vi "Show UI For Selection.vi"(8 "Error In":errorcluster, 11 "Pane Relief Main UI in":refnum<class "Pane Relief Main UI.lvclass">) -> (0 "Error Out":errorcluster, 3 "Pane Relief Main UI out":refnum<class "Pane Relief Main UI.lvclass">)   [LabVIEW 2017, in "Pane Relief Main UI.lvlib" / "Pane Relief Main UI.lvclass"]
uses:
  Pane Relief Main UI.lvclass
  Pane Relief Main UI.lvclass/Pane Relief Main UI.ctl
  Panel Object Actions UI/Panel Object Actions UI Messages/Show Panel Object Actions UI Msg/Show Panel Object Actions UI Msg.lvclass/Show Panel Object Actions UI Msg.ctl
  <vilib>/ActorFramework/Message Enqueuer/Message Enqueuer.lvclass/Message Enqueuer.ctl
  <vilib>/ActorFramework/Message Enqueuer/Enqueue.vi
  Panel Object Actions UI/Panel Object Actions UI Messages/Show Panel Object Actions UI Msg/Show Panel Object Actions UI Msg.lvclass
  C:/Program Files (x86)/National Instruments/LabVIEW 2017/vi.lib/ActorFramework/Message/Message.lvclass
  <vilib>/ActorFramework/Message Priority Queue/Priority Enqueue.vi
  Panel Object/Panel Object.lvclass
  <vilib>/MNProjects/Panel Manager/panel-actors/Source/Panel Actor Messages/Show Panel Msg/Show Panel Msg.lvclass
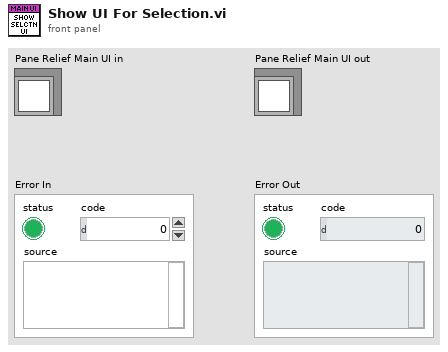
[diagram p1: front panel]
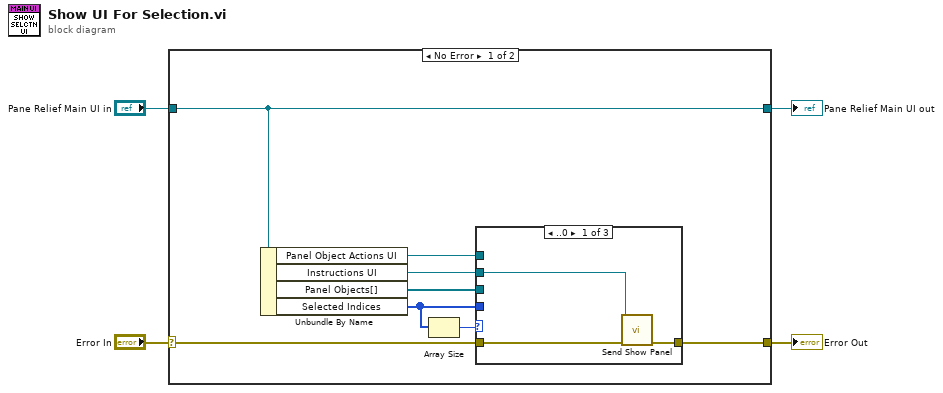
[diagram p0: block diagram]
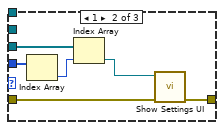
[diagram p2: hidden frame]
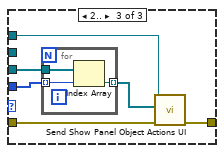
[diagram p3: hidden frame]
diagram:
  n1 = case shown="No Error" "Error In" {
    selector: "Error In" -> [w10 w32]
    tunnel: [w9 w32] -> w1
    tunnel: [w11 w31] -> w3
    tunnel: "Pane Relief Main UI in" -> [w11 w31]
    frame No Error {
      n2 = Unbundle By Name(w11) -> ("Panel Object Actions UI"=w6:refnum<class "Message Enqueuer.lvclass">, "Instructions UI"=w7:refnum<class "Message Enqueuer.lvclass">, "Panel Objects[]"=w12:refnum<class "Panel Object.lvclass">[], "Selected Indices"=w5:i32[])
      n3 = Array Size(array=w5) -> (size(s)=w8:i32)
      n4 = case shown="..0" w8 {
        tunnel: w12 -> [_ w21 w24]
        tunnel: w10 -> [w14 w19 w26]
        tunnel: [w15 w18 w27] -> w9
        tunnel: w7 -> [w13 _ _]
        tunnel: w6 -> [_ _ w25]
        tunnel: w5 -> [_ w17 w22]
        frame ..0 {
          n5 = call <vilib>:"Send Show Panel.vi"("error in (no error)"=w14, "Message Enqueuer in"=w13) -> ("error out"=w15:errorcluster)  [unwired: 8 in, 1 out]
        }
        frame 1 {
          n6 = Index Array(array=w17) -> (element=w16:i32)  [unwired: 1 in]
          n7 = Index Array(array=w21, index=w16) -> (element=w20:refnum<class "Panel Object.lvclass">)
          n8 = call-dynamic "Show Settings UI.vi"("Error In"=w19, "Panel Object in"=w20) -> ("Error Out"=w18:errorcluster)  [unwired: 8 in, 1 out]
        }
        frame 2.. {
          n9 = for {
            tunnel: w24 -> [w30]
            tunnel: [w29] -> w23 mode=indexing
            tunnel: w22 -> [w28] mode=indexing
            n10 = Index Array(array=w30, index=w28) -> (element=w29:refnum<class "Panel Object.lvclass">)
          }
          n11 = call "Send Show Panel Object Actions UI.vi"("error in (no error)"=w26, "Panel Objects"=w23, "Message Enqueuer"=w25) -> ("error out"=w27:errorcluster)  [unwired: 7 in, 1 out]
        }
      }
    }
    frame Error {
    }
  }
  "Pane Relief Main UI out" <- w3
  "Error Out" <- w1
